vi "Export Configuration RTM.vi"(8 "error in (no error)":errorcluster, 11 "Node Ptr":u64 format="%.0x") -> (0 "error out":errorcluster)   [LabVIEW 2020, in "Routing and Faulting System Explorer.lvlib"]
uses:
  Routing and Faulting System Explorer.lvlib
  Scripting/Routing and Faulting Scripting.lvlib
panel:
  in  "Tag":string
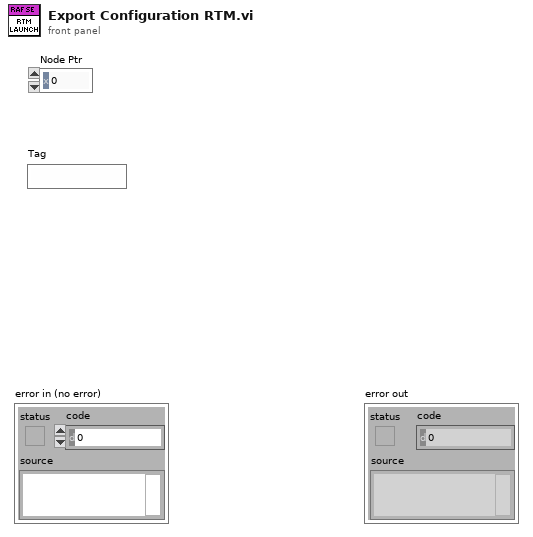
[diagram p1: front panel]
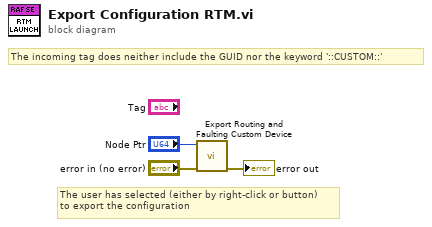
[diagram p0: block diagram]
diagram:
  # "The user has selected (either by right-click or button)\nto export the configuration"
  # "The incoming tag does neither include the GUID nor the keyword '::CUSTOM::'"
  n1 = call "Export Routing and Faulting Custom Device.vi"("error in"="error in (no error)", "routing and faulting custom device in"="Node Ptr") -> ("error out"=→"error out":errorcluster)  [unwired: 8 in, 1 out]
